vi "Tabelle erstellen.vi"() -> (3 "Tabelle":T2[][](array[typedef]))   [LabVIEW 2020, in "EPA 1065.lvlib" / "Interference verificaton 1065-375.lvlib"]
uses:
  Interference verificaton 1065-375.lvlib
  Visualisierungs Elemente/String - Ausgabefeld.ctl
  Modus.ctl
  Aktion FGV Interference.ctl
  Seiten/FT-IR/FGV FT-IR Gasliste Aktionen.ctl
  Aktion Index uebersetzten.ctl
  Sprachverwaltung/FGV Aktion Tabelle zerlegen.ctl
  Seiten/FT-IR/FT-IR.lvlib
  Allgemein/allgemeine Sub-VIs.lvlib
  Sprachverwaltung/Sprachverwaltung.lvlib
panel:
  in  "Modus 2":T1 caption="Modus:" items=["Messen", "CG zu Entnahmestelle"]
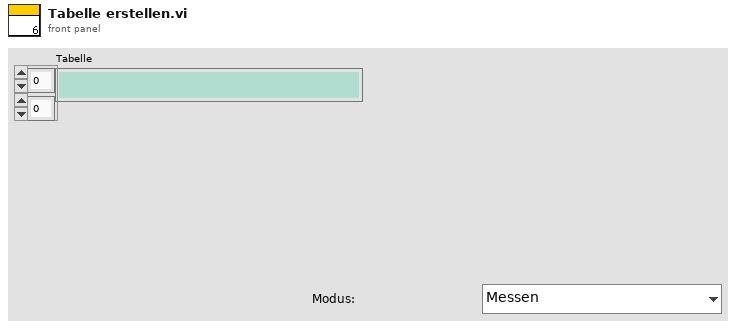
[diagram p1: front panel]
types:
  T1 = typedef "EPA 1065.lvlib/Interference verificaton 1065-375.lvlib/Modus.ctl" = u16
  T2 = typedef "String - Ausgabefeld.ctl" = string
  T3 = typedef "Sprachverwaltung.lvlib/FGV Aktion Tabelle zerlegen.ctl" = enum16{"laden", "vereinzeln", "speichern"}
  T4 = typedef "EPA 1065.lvlib/Interference verificaton 1065-375.lvlib/Aktion Index uebersetzten.ctl" = enum16{"lesen", "schreiben", "auswerten"}
  T5 = typedef "FT-IR.lvlib/FGV FT-IR Gasliste Aktionen.ctl" = enum16{"lesen", "Gasliste FT-IR", "Gasliste ausgelesen", "laden", "speichern", "löschen"}
  T6 = typedef "EPA 1065.lvlib/Interference verificaton 1065-375.lvlib/Aktion FGV Interference.ctl" = enum16{"Lesen", "TestKonfig", "TestSetting", "Einheiten", "Ergebnis", "Laden", "Tabelle", "Speichern", "löschen"}
  T7 = typedef "EPA 1065.lvlib/Interference verificaton 1065-375.lvlib/TestKonfig.ctl" = cluster{"Komponente:":u16, "Modus":T1, "CG Aufschaltzeit:":dbl, "Interferent 1:":u16, "Interferent 2:":u16, "Interferent 3:":u16, "Gasflaschen Nr.:":string, "Gasflaschen Nr.: 2":string, "Gasflaschen Nr.: 3":string, "Inter 1 aktiv":bool, "Inter 2 aktiv":bool, "Inter 3 aktiv":bool, "Accuracy":string, "Accuracy 2":string, "Accuracy 3":string, "Konzentration 1:":dbl, "Konzentration 2:":dbl, "Konzentration 3:":dbl}
  T8 = typedef "EPA 1065.lvlib/Interference verificaton 1065-375.lvlib/Ergebnis.ctl" = cluster{"Interferent 1":sgl, "Interferent 2":sgl, "Interferent 3":sgl, "Interferent 4":sgl, "Komponente 1":sgl, "Komponente 2":sgl, "Komponente 3":sgl}
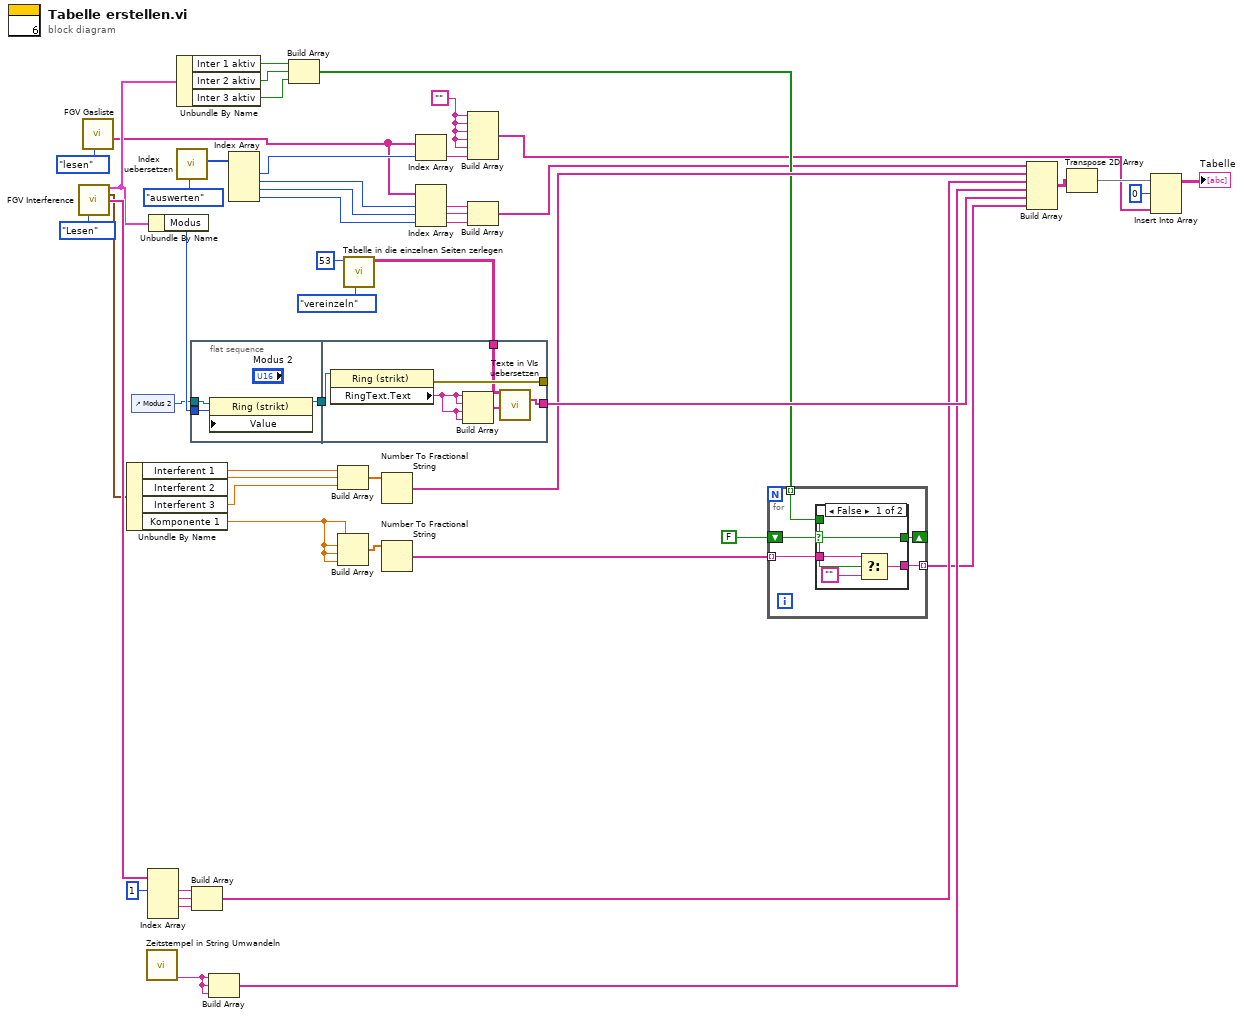
[diagram p0: block diagram]
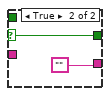
[diagram p2: hidden frame]
diagram:
  w12 = ""
  n1 = call "FGV Interference.vi"("Aktion FGV Interference"=Aktion_FGV_Interference."Lesen") -> ("TestKonfig 2"=w31:T7, "Ergebnis"=w39:T8, "Êinheiten"=w40:string[])  [unwired: 9 in, 3 out]
  n2 = call "FGV Gasliste.vi"("Aktionen"=FGV_FT-IR_Gasliste_Aktionen."lesen") -> ("Aktuelle Gasliste gesamt"=w17:T2[])  [unwired: 8 in, 2 out]
  n3 = Unbundle By Name(w39) -> ("Interferent 1"=w42:sgl, "Interferent 2"=w43:sgl, "Interferent 3"=w44:sgl, "Komponente 1"=w24:sgl)
  n4 = control-ref of="Modus 2"() -> (w27:refnum<vi>)
  n5 = call "Zeitstempel in String Umwandeln.vi"() -> ("Zeitstempel"=w34:string)  [unwired: 10 in, 1 out]
  n6 = Index Array(array=w40, index #1=1 ("Index")) -> (element #1=w10:string, element #2=w9:string, element #3=w8:string)  [unwired: 3 in, 1 out]
  n7 = Unbundle By Name(w31) -> ("Modus"=w49:T1)
  n8 = Unbundle By Name(w31) -> ("Inter 1 aktiv"=w30:bool, "Inter 2 aktiv"=w29:bool, "Inter 3 aktiv"=w28:bool)
  n9 = call "Index uebersetzen.vi"("Aktion"=Aktion_Index_uebersetzten."auswerten") -> ("Komponenten"=w25:i32[])  [unwired: 9 in, 1 out]
  n10 = flat-sequence {
    tunnel: w49 -> [w54]
    tunnel: [w53] -> w36
    tunnel: w27 -> [w52]
    tunnel: [w60] -> _
    tunnel: [w56] -> w50
    tunnel: w36 -> [w59]
    tunnel: w1 -> [w55]
    frame #0 {
      n11 = property class="Ring (strikt)"(reference=w52, "Value"=w54) -> (reference out=w53:refnum<vi>)  [unwired: 1 in, 1 out]
    }
    frame #1 {
      n12 = property on="Eigenschaftsknoten" class="Ring (strikt)"(reference=w59) -> (error out=w60:errorcluster, "RingText.Text"=w58:string)  [unwired: 1 in, 1 out]
      n13 = Build Array(w58, w58, w58, w58) -> (w57:string[])
      n14 = call "Texte in VIs uebersetzen.vi"("Sprachliste"=w55, "String-Array zum Übersetzen"=w57) -> ("String-Array zum Übersetzen"=w56:string[])  [unwired: 9 in, 4 out]
    }
  }
  n15 = Build Array(w10, w9, w8) -> (w47:string[])
  n16 = Build Array(w34, w34, w34) -> (w48:string[])
  n17 = Index Array(array=w25) -> (element #1=w21:i32, element #2=w6:i32, element #3=w5:i32, element #4=w4:i32)  [unwired: 4 in]
  n18 = Build Array(w30, w29, w28) -> (w23:bool[])
  n19 = Build Array(w42, w43, w44) -> (w45:sgl[])
  n20 = Build Array(w24, w24, w24, w24) -> (w35:sgl[])
  n21 = call "Tabelle in die einzelnen Seiten zerlegen.vi"("Aktion"=FGV_Aktion_Tabelle_zerlegen."vereinzeln", "Index (Seite)"=53) -> ("Sprachliste"=w1:string[][])  [unwired: 7 in, 2 out]
  n22 = Number To Fractional String(number=w45) -> (F-format string=w46:string[])  [unwired: 3 in]
  n23 = Number To Fractional String(number=w35) -> (F-format string=w33:string[])  [unwired: 3 in]
  n24 = Index Array(array=w17, index=w21) -> (element=w41:T2)
  n25 = Index Array(array=w17, index #1=w6, index #2=w5, index #3=w4) -> (element #1=w20:T2, element #2=w19:T2, element #3=w18:T2)
  n26 = Build Array(w12, w12, w12, w12, w12, w41) -> (w14:T2[])
  n27 = Build Array(w20, w19, w18) -> (w16:T2[])
  n28 = for {
    tunnel: w33 -> [w64] mode=indexing
    tunnel: [w65] -> w32 mode=indexing
    tunnel: w23 -> [w63] mode=indexing
    shift-right: [w61] -> _
    shift-left: FALSE -> [w62]
    n29 = case shown="False" w62 {
      selector: w62 -> [_ w71]
      tunnel: [w69 ""] -> w65
      tunnel: w64 -> [w68 _]
      tunnel: w63 -> [w66 _]
      tunnel: [w66 w71] -> w61
      frame False {
        n30 = Select(t=w68, s=w66, f="") -> (s? t:f=w69:string)
      }
      frame True {
      }
    }
  }
  n31 = Build Array(w16, w46, w47, w48, w50, w32) -> (w51:T2[][])
  n32 = Transpose 2D Array(2D array=w51) -> (transposed array=w15:T2[][])
  n33 = Insert Into Array(array=w15, index (row)=0 ("Index (Zeile)"), new element=w14) -> (→"Tabelle":T2[][])  [unwired: 1 in]
